vi "Rosie_Control_Panel.vi"(11 "IP Address of Remote Device":string="196.254.31.204") -> ()   [LabVIEW 2020]
panel:
  out "TCP Close ms":u32
  out "TCP Open ms":u32
  out "Gettable Get, ms":u32(graph)
  out "Settable Get, ms":u32(graph)
  in  "Zero Time":bool
  out "Settable Device Keywords":string[](array[string])
  out "Live Readback Values":string[](array[string])
  in  "Set All":bool
  in  "Set Values\n(Fully empty cells will not be set)":string[](array[string])
  out "Live Responses":string[](array[string])
  out "Non-Settable Device Keywords":string[](array[string])
  in  "Disconnect":bool
  # "\"Rosie\" Device Control Panel"
  # "Rosie rivets together the trigger system with various non-trigger-counting diagnostics."
  # "VI Instructions\n\n1. Make sure you know the Device IP Address.\n2. From Windows command prompt, confirm ping to IP address.\n3. Type the correct device IP address into this VI.\n3. Run this VI. *Note:* Only one TCP connection to the device's SCPI-like server can run at a time.\n4. When finished, disconnect safely from the device via the \"Disconnect\" toggle button. (Not the Abort button).\n\nCreated by Scott Feister on July 25, 2022."
  # "Settings *ARE NOT SAVED TO DEVICE* and are lost on device reset! Write them down!"
  # "1. Resets the trigger count to zero.\n2. Transmits this system's current time."
  # "Network debugging ONLY: TCP Latency (added Sep 2022)"
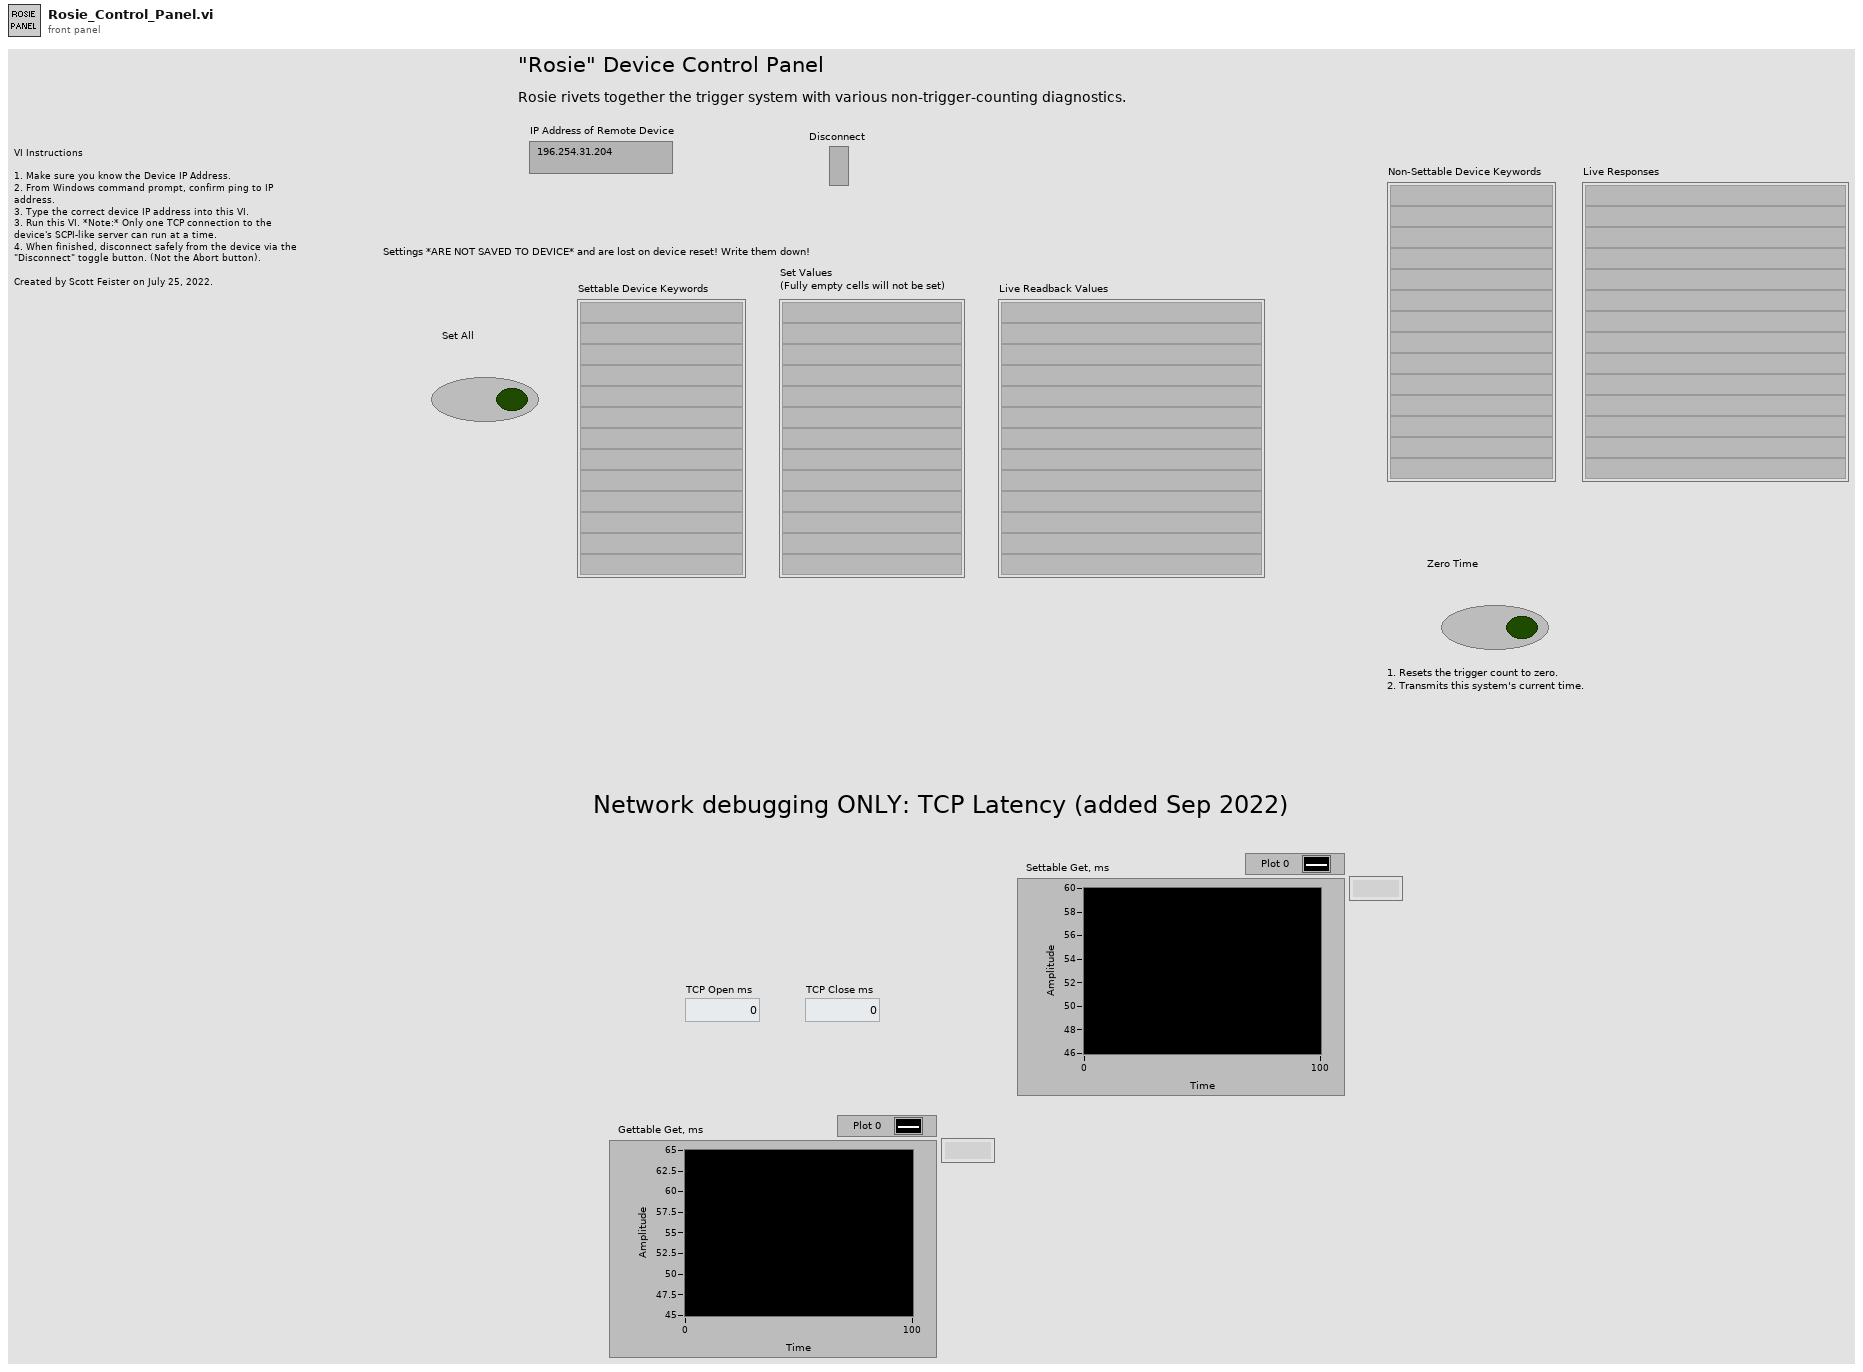
[diagram p1: front panel]
types:
  T1 = typedef "DDAQ-Keyword.ctl" = cluster{"Keyword":string, "Gettable":bool, "Settable":bool, "Is Array":bool, "Data Type":string, "Description":string}
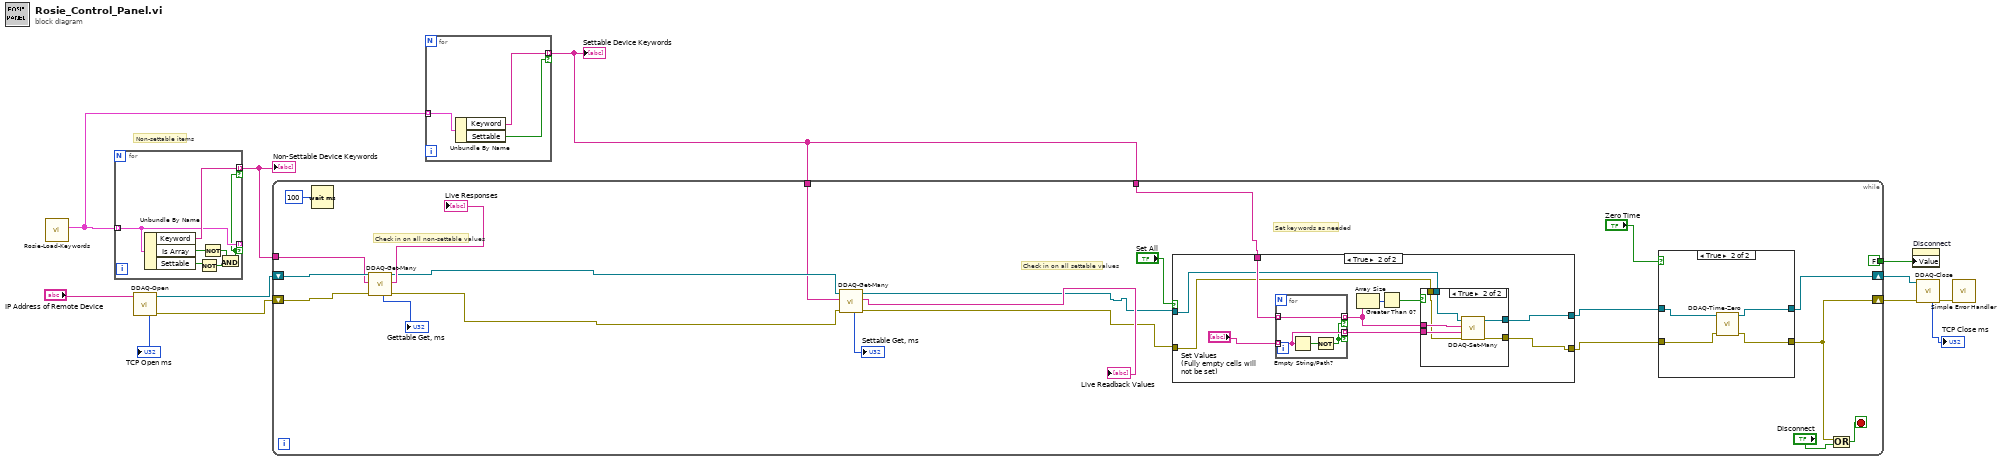
[diagram p0: block diagram]
diagram:
  # "Non-settable items"
  n1 = call "Rosie-Load-Keywords.vi"() -> ("Diodes Keywords Array"=w5:T1[])  [unwired: 11 in]
  n2 = for {
    tunnel: w5 -> [w17] mode=indexing
    tunnel: [w19] -> w2 mode=indexing if=w13
    tunnel: [w17] -> _ mode=indexing if=w13
    n3 = Unbundle By Name(w17) -> ("Keyword"=w19:string, "Is Array"=w18:bool, "Settable"=w16:bool)
    n4 = Not(x=w16) -> (.not. x?=w15:bool)
    n5 = Not(x=w18) -> (.not. x?=w14:bool)
    n6 = And(x=w14, y=w15) -> (x .and. y?=w13:bool)
  }
  "Non-Settable Device Keywords" <- w2
  n7 = call "DDAQ-Open.vi"("IP Address of Nucleo Device"="IP Address of Remote Device") -> ("error out"=w11:errorcluster, "connection ID"=w12:refnum<k5>, "Elapsed time, ms (debug)"=→"TCP Open ms":u32)  [unwired: 8 in]
  n8 = for {
    tunnel: w5 -> [w21] mode=indexing
    tunnel: [w22] -> w1 mode=indexing if=w20
    n9 = Unbundle By Name(w21) -> ("Keyword"=w22:string, "Settable"=w20:bool)
  }
  "Settable Device Keywords" <- w1
  n10 = while {
    shift-right: [w40] -> w10
    shift-left: w12 -> [w38]
    shift-right: [w39] -> w9
    shift-left: w11 -> [w36]
    tunnel: [FALSE] -> w7
    tunnel: w1 -> [w25]
    tunnel: w2 -> [w37]
    tunnel: w1 -> [w29]
    stop <- w42 stop-if-true
    # "Set keywords as needed"
    # "Check in on all settable values"
    # "Check in on all non-settable values"
    n11 = Wait (ms)(milliseconds to wait=u32 100) -> ()  [unwired: 1 out]
    n12 = call "DDAQ-Get-Many.vi"("error in (no error)"=w36, "SCPI-like Keywords (leave off question marks)"=w37, "connection ID"=w38) -> ("error out"=w32:errorcluster, "Responses"=→"Live Responses":string[], "connection ID out"=w33:refnum<k5>, "Elapsed time, ms (debug)"=→"Gettable Get, ms":u32)  [unwired: 4 in, 1 out]
    n13 = call "DDAQ-Get-Many.vi"("error in (no error)"=w32, "SCPI-like Keywords (leave off question marks)"=w29, "connection ID"=w33) -> ("error out"=w27:errorcluster, "Responses"=→"Live Readback Values":string[], "connection ID out"=w28:refnum<k5>, "Elapsed time, ms (debug)"=→"Settable Get, ms":u32)  [unwired: 4 in, 1 out]
    n14 = case shown="True" "Set All" {
      tunnel: w25 -> [_ w57]
      tunnel: w28 -> [w46 w53]
      tunnel: w27 -> [w47 w52]
      tunnel: [w47 w49] -> w23
      tunnel: [w46 w50] -> w24
      frame False {
      }
      frame True {
        n15 = for {
          tunnel: "Set Values\n(Fully empty cells will not be set)" -> [w67] mode=indexing
          tunnel: w57 -> [w68] mode=indexing
          tunnel: [w68] -> w55 mode=indexing if=w66
          tunnel: [w67] -> w54 mode=indexing if=w66
          n16 = Empty String/Path?(string/path=w67) -> (empty?=w69:bool)
          n17 = Not(x=w69) -> (.not. x?=w66:bool)
        }
        n18 = Array Size(array=w55) -> (size(s)=w56:i32)
        n19 = Greater Than 0?(x=w56) -> (x > 0?=w51:bool)
        n20 = case shown="True" w51 {
          tunnel: w55 -> [_ w65]
          tunnel: w54 -> [_ w64]
          tunnel: w53 -> [w59 w63]
          tunnel: w52 -> [w58 w62]
          tunnel: [w59 w61] -> w50
          tunnel: [w58 w60] -> w49
          frame False {
          }
          frame True {
            n21 = call "DDAQ-Set-Many.vi"("error in (no error)"=w62, "Set Values"=w64, "SCPI-like Keywords (leave off space, value)"=w65, "connection ID"=w63) -> ("error out"=w60:errorcluster, "connection ID out"=w61:refnum<k5>)  [unwired: 5 in, 1 out]
          }
        }
      }
    }
    n22 = case shown="True" "Zero Time" {
      tunnel: w24 -> [w70 w75]
      tunnel: [w71 w72] -> w39
      tunnel: w23 -> [w71 w73]
      tunnel: [w70 w74] -> w40
      frame False {
      }
      frame True {
        n23 = call "DDAQ-Time-Zero.vi"("error in (no error)"=w73, "connection ID"=w75) -> ("error out"=w72:errorcluster, "connection ID out"=w74:refnum<k5>)  [unwired: 8 in]
      }
    }
    n24 = Or(x=w39, y="Disconnect") -> (x .or. y?=w42:bool)
  }
  n25 = property on="Disconnect" class="Bool (strict)"("Value"=w7) -> ()  [unwired: 2 in, 2 out]
  n26 = call "DDAQ-Close.vi"("error in (no error)"=w9, "connection ID"=w10) -> ("error out"=w8:errorcluster, "Elapsed time, ms (debug)"=→"TCP Close ms":u32)  [unwired: 8 in]
  n27 = call <vilib>:"Simple Error Handler.vi"("error in (no error)"=w8) -> ()  [unwired: 4 in, 5 out]
